vi "Configure Measurement.vi"(0 "VISA resource name":refnum<visa-resource-name>, 1 "Enable Range (T: Enable)":bool=TRUE, 5 "Measurement Function (0: DC Volts)":u16(ring) items=["DC Volts", "AC Volts", "DC Current", "AC Current", "2-Wire Resistance", "4-Wire Resistance", "Frequency", "AC and DC rms Current", "AC and DC rms Volts", "Continuity", "Diode"], 7 "Measurement Rate (0: Slow)":u16(ring) items=["Slow", "Medium", "Fast"], 9 "Decibel Reference Impedance (1: 2 Ohms)":u16(ring)=1 items=["2 Ohms"=1, "4 Ohms"=2, "8 Ohms"=3, "16 Ohms"=4, "50 Ohms"=5, "75 Ohms"=6, "93 Ohms"=7, "110 Ohms"=8, "124 Ohms"=9, "125 Ohms"=10, "135 Ohms"=11, "150 Ohms"=12, "250 Ohms"=13, "300 Ohms"=14, "500 Ohms"=15, "600 Ohms"=16, "800 Ohms"=17, "900 Ohms"=18, "1000 Ohms"=19, "1200 Ohms"=20, "8000 Ohms"=21], 11 "error in (no error)":errorcluster, 12 "Measurement Modifier (0: None)":u16(ring) items=["None", "Decibels", "Decibel Power"], 13 "Manual Range (1: 200 mV, 200 Ohms, 20 mA AC, 2 kHz, 200 miuA DC)":u16(ring)=1 items=["200 mV, 200 Ohms, 20 mA AC, 2 kHz, 200 miuA DC"=1, " 2 V, 2 kOhms, 200 mA AC, 20 kHz, 2000 miuA DC"=2, "20 V, 20 kOhms, 2 A AC, 200 kHz, 20 mA DC"=3, "200 V, 200 kOhms, 10 A AC, 1000 kHz, 200 mA DC"=4, "1000 V DC, 2 MOhms, 2 A DC"=5, "20 MOhms, 10 A DC"=6, "100 MOhms"=7]) -> (4 "VISA resource name out":refnum<visa-resource-name>, 15 "error out":errorcluster)   [LabVIEW 2015, in "Fluke 8808.lvlib"]
doc: "Configures the measurement type, resolution, and range on the instrument."
uses:
  <instrlib>/Fluke 8808/Fluke 8808.lvlib
panel:
  # "Voltage Measurement Function"
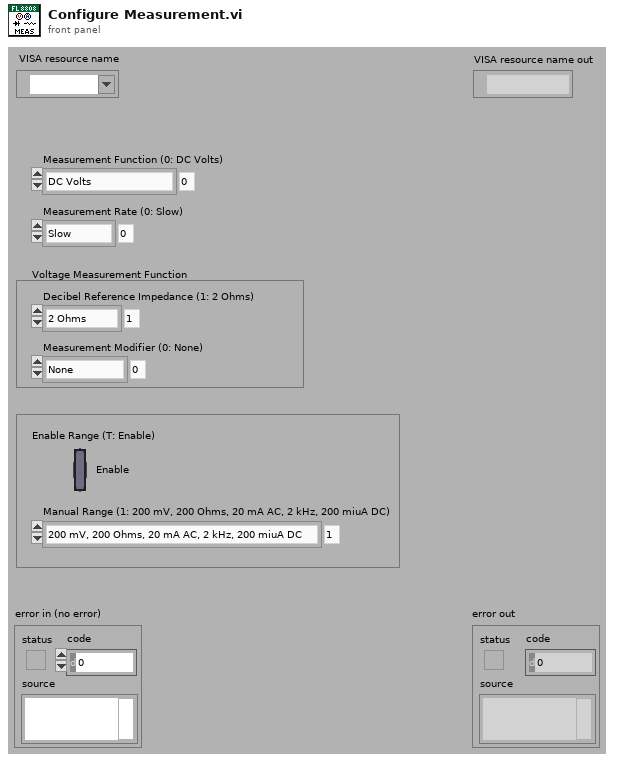
[diagram p1: front panel]
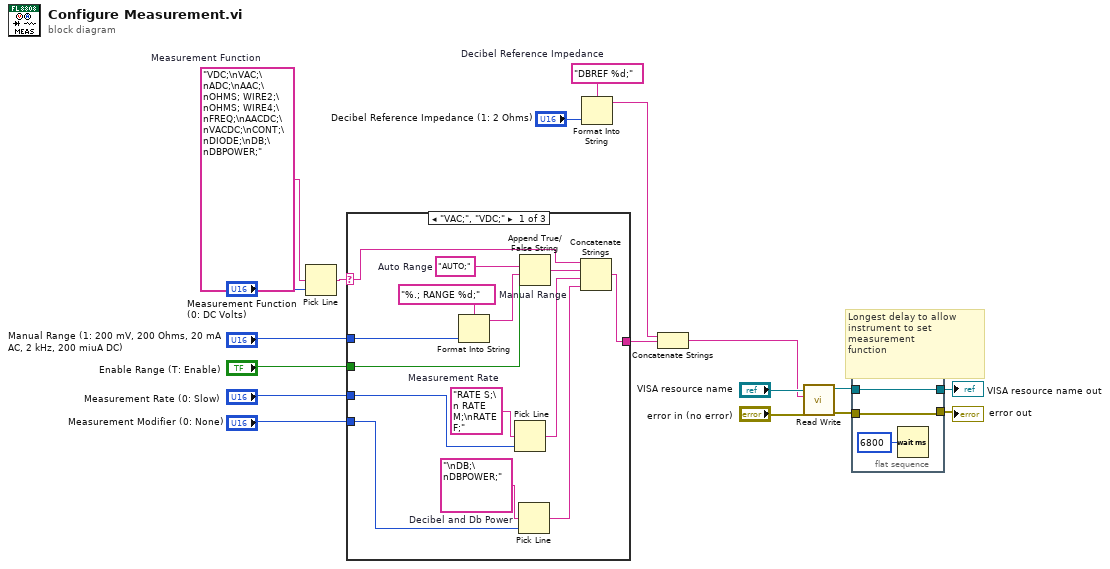
[diagram p0: block diagram]
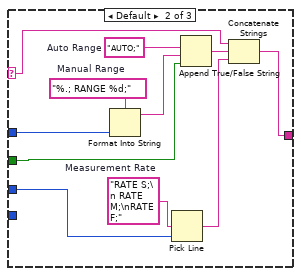
[diagram p2: hidden frame]
diagram:
  w10 = "DBREF %d;"  # Decibel Reference Impedance
  w12 = "VDC;\nVAC;\nADC;\nAAC;\nOHMS; WIRE2;\nOHMS; WIRE4;\nFREQ;\nAACDC;\nVACDC;\nCONT;\nDIODE;\nDB;\nDBPOWER;"  # Measurement Function
  # "Longest delay to allow \ninstrument to set\nmeasurement \nfunction"
  n1 = Pick Line(multi-line string=w12, line index="Measurement Function (0: DC Volts)") -> (output string=w11:string)  [unwired: 1 in]
  n2 = case shown="\"VAC;\", \"VDC;\"" w11 {
    selector: w11 -> [w19 w33 w44]
    tunnel: "Manual Range (1: 200 mV, 200 Ohms, 20 mA AC, 2 kHz, 200 miuA DC)" -> [w23 w37 _]
    tunnel: "Enable Range (T: Enable)" -> [w22 w36 _]
    tunnel: [w24 w34 w44] -> w8
    tunnel: "Measurement Rate (0: Slow)" -> [w21 w35 _]
    tunnel: "Measurement Modifier (0: None)" -> [w20 _ _]
    frame "VAC;", "VDC;" {
      w26 = "\nDB;\nDBPOWER;"  # Decibel and Db Power
      w28 = "RATE S;\n RATE M;\nRATE F;"  # Measurement Rate
      w30 = "AUTO;"  # Auto Range
      w32 = "%.; RANGE %d;"  # Manual Range
      n3 = Format Into String(format string=w32, w23) -> (resulting string=w31:string)  [unwired: 2 in, 1 out]
      n4 = Pick Line(multi-line string=w28, line index=w21) -> (output string=w29:string)  [unwired: 1 in]
      n5 = Pick Line(multi-line string=w26, line index=w20) -> (output string=w25:string)  [unwired: 1 in]
      n6 = Append True/False String(1:w22, 2:w31, 3:w30) -> (0:w27:string)  [unwired: 1 in]
      n7 = Concatenate Strings(w19, w27, w29, w25) -> (w24:string)
    }
    frame Default {
      w39 = "RATE S;\n RATE M;\nRATE F;"  # Measurement Rate
      w41 = "AUTO;"  # Auto Range
      w43 = "%.; RANGE %d;"  # Manual Range
      n8 = Format Into String(format string=w43, w37) -> (resulting string=w42:string)  [unwired: 2 in, 1 out]
      n9 = Pick Line(multi-line string=w39, line index=w35) -> (output string=w40:string)  [unwired: 1 in]
      n10 = Append True/False String(1:w36, 2:w42, 3:w41) -> (0:w38:string)  [unwired: 1 in]
      n11 = Concatenate Strings(w33, w38, w40) -> (w34:string)
    }
    frame "CONT;", "DIODE;" {
    }
  }
  n12 = Format Into String(format string=w10, "Decibel Reference Impedance (1: 2 Ohms)") -> (resulting string=w9:string)  [unwired: 2 in, 1 out]
  n13 = Concatenate Strings(w9, w8) -> (w7:string)
  n14 = call <instrlib>:"Read Write.vi"("error in (no error)"="error in (no error)", "Write String"=w7, "VISA resource name"="VISA resource name") -> ("error out"=w13:errorcluster, "VISA resource name out"=w14:refnum<visa-resource-name>)  [unwired: 6 in, 1 out]
  n15 = flat-sequence {
    tunnel: w14 -> [w47]
    tunnel: [w47] -> w16
    tunnel: [w46] -> w15
    tunnel: w13 -> [w46]
    frame #0 {
      n16 = Wait (ms)(milliseconds to wait=u32 6800) -> ()  [unwired: 1 out]
    }
  }
  "error out" <- w15
  "VISA resource name out" <- w16
